vi "Set Limits.vi"(0 "reference in":refnum<class "Simulated-PowerModule.lvclass">, 5 "Limits":T1, 11 "Error In":errorcluster) -> (4 "reference out":refnum<class "Simulated-PowerModule.lvclass">, 15 "Error Out":errorcluster)   [LabVIEW 2023, in "Simulated-PowerModule.lvlib" / "Simulated-PowerModule.lvclass"]
uses:
  Simulated-PowerModule.lvclass
  builds/PowerModuleInterface/home/lvuser/natinst/bin/PowerModuleInterface.lvlibp/Classes/PowerModule_interface/Limits.ctl
  builds/PowerModuleInterface/home/lvuser/natinst/bin/PowerModuleInterface.lvlibp/Classes/PowerModule_interface/PowerModuleInterface.lvclass
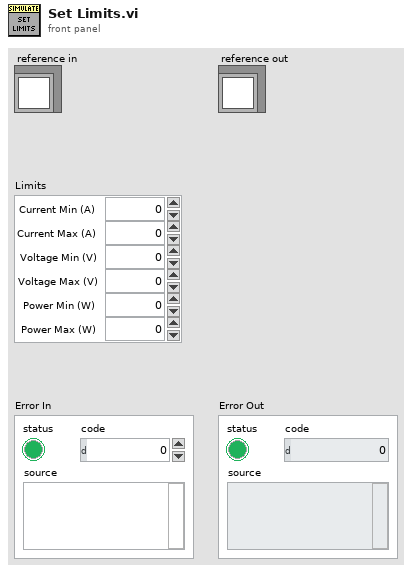
[diagram p1: front panel]
types:
  T1 = typedef "PowerModuleInterface.lvlibp/PowerModuleInterface.lvclass/Limits.ctl" = cluster{"Current Max (A)":dbl, "Current Min (A)":dbl, "Voltage Max (V)":dbl, "Voltage Min (V)":dbl, "Power Max (W)":dbl, "Power Min (W)":dbl}
  T2 = typedef "Simulated-PowerModule.lvlib/Simulated-PowerModule.lvclass/ObjectAttributes.ctl" = cluster{"JSON Config Path":path, "Configuration":T3, "connected":bool, "reserved":bool, "energized":bool, "output enabled":bool, "Mode":T4, "Range":T5, "Slew Rates":T6, "Setpoints":cluster{"voltage":dbl, "current":dbl, "resistance":dbl}, "Measurements":cluster{"voltage":dbl, "current":dbl, "resistance":dbl}, "Limits":T1, "active faults":string[], "fault":bool, "profile":dbl[][], "step dt":i64}
  T3 = typedef "Simulated-PowerModule.lvlib/Simulated-PowerModule.lvclass/Configuration.ctl" = cluster{"IP Address":string}
  T4 = typedef "Simulated-PowerModule.lvlib/Simulated-PowerModule.lvclass/Mode.ctl" = u16
  T5 = typedef "PowerModuleInterface.lvlibp/PowerModuleInterface.lvclass/Range.ctl" = cluster{"Current Max (A)":dbl, "Current Min (A)":dbl, "Voltage Max (V)":dbl, "Voltage Min (V)":dbl}
  T6 = typedef "PowerModuleInterface.lvlibp/PowerModuleInterface.lvclass/Slew Rates.ctl" = cluster{"Current Decrease (A/sec)":dbl, "Current Increase (A/sec)":dbl, "Voltage Decrease (V/sec)":dbl, "Voltage Increase (V/sec)":dbl, "Resistance Decrease (Ohm/sec)":dbl, "Resistance Increase (Ohm/sec)":dbl}
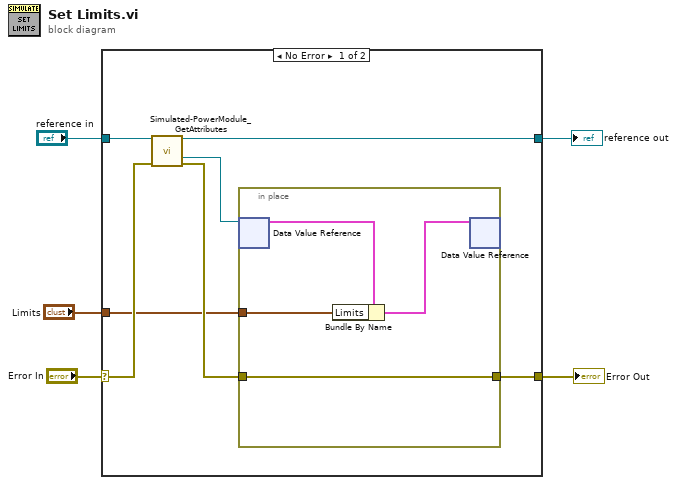
[diagram p0: block diagram]
diagram:
  n1 = case shown="No Error" "Error In" {
    selector: "Error In" -> [w12 w18]
    tunnel: [w8 w17] -> w5
    tunnel: [w9 w18] -> w3
    tunnel: "reference in" -> [w7 w17]
    tunnel: "Limits" -> [w6 _]
    frame No Error {
      n2 = call "Simulated-PowerModule_GetAttributes.vi"("reference in"=w7, "Error In"=w12) -> ("reference out"=w8:refnum<class "Simulated-PowerModule.lvclass">, "DataRef"=w11:refnum<data-value>, "Error Out"=w10:errorcluster)  [unwired: 10 in, 1 out]
      n3 = in-place {
        in-place-border: w10 -> [w14]
        in-place-border: [w14] -> w9
        in-place-border: w6 -> [w13]
        n4 = in-place-dvr #1(w11) -> (w15:T2)  [unwired: 1 out]
        n5 = Bundle By Name(cluster=w15, "Limits"=w13) -> (w16:T2)
        n6 = in-place-dvr #1(w16) -> ()  [unwired: 2 out]
      }
    }
    frame Error {
    }
  }
  "Error Out" <- w3
  "reference out" <- w5
